vi "movestageparams.vi"(1 "Params in":T1, 2 "command":string) -> (0 "Params out":T1)   [LabVIEW 2015]
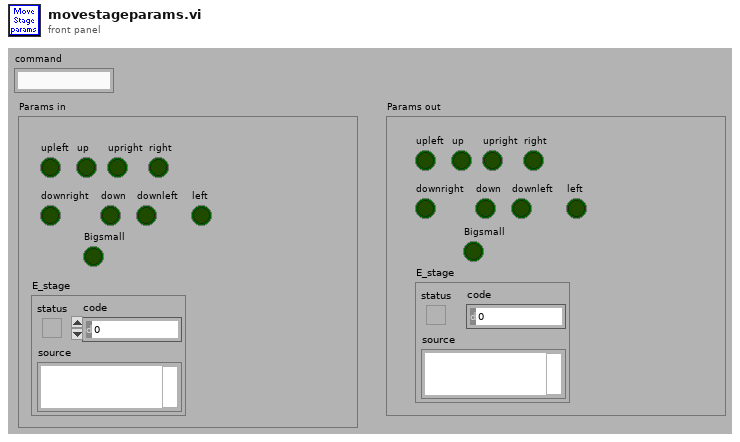
[diagram p1: front panel]
types:
  T1 = cluster{"upleft":bool, "up":bool, "upright":bool, "right":bool, "downright":bool, "down":bool, "downleft":bool, "left":bool, "Bigsmall":bool, "E_stage":errorcluster}
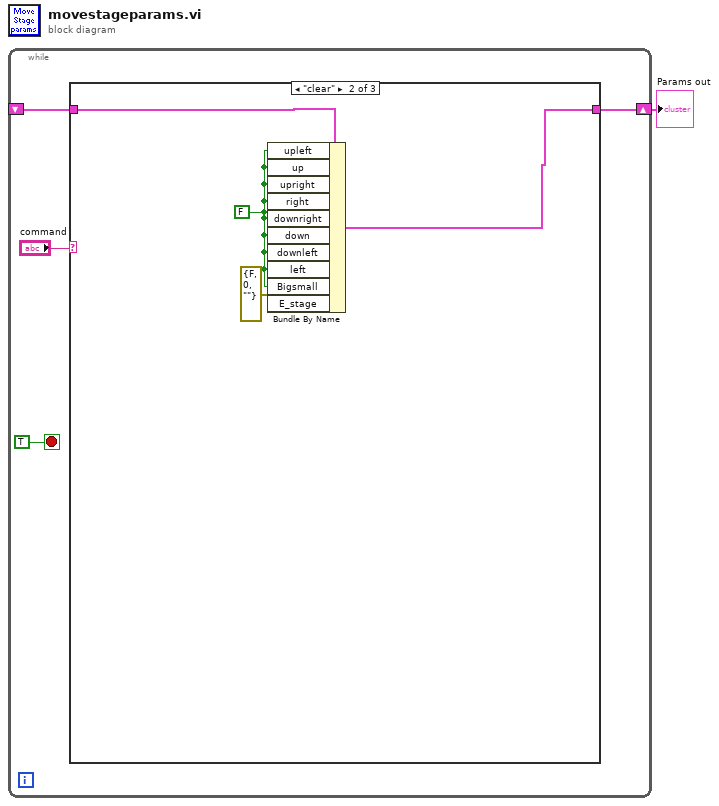
[diagram p0: block diagram]
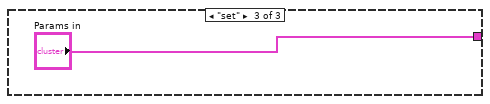
[diagram p3: hidden frame]
diagram:
  n1 = while {
    shift-right: [w3] -> w1
    shift-left: _ -> [w2]
    stop <- TRUE stop-if-true
    n2 = case shown="\"clear\"" "command" {
      tunnel: [w6 w9 "Params in"] -> w3
      tunnel: w2 -> [w6 w10 _]
      frame "get", Default {
      }
      frame "clear" {
        w8 = FALSE ("upleft")
        n3 = Bundle By Name(cluster=w10, "upleft"=w8, "up"=w8, "upright"=w8, "right"=w8, "downright"=w8, "down"=w8, "downleft"=w8, "left"=w8, "Bigsmall"=w8, "E_stage"=errorcluster {"status"=FALSE, "code"=0, "source"=""}) -> (w9:T1)
      }
      frame "set" {
      }
    }
  }
  "Params out" <- w1
